vi "ZMC Open Eth.vi"(8 "error in (no error)":errorcluster caption="错误输入（无错误）", 10 "phandle":u32, 11 "ipaddr":string) -> (0 "error out":errorcluster caption="错误输出", 1 "function return":i32, 2 "phandle out":u32, 3 "ipaddr out":string)   [LabVIEW 2019, in "zauxdll.lvlib"]
doc: "int32 __stdcall ZMC_OpenEth(char *ipaddr, ZMC_HANDLE * phandle);"
uses:
  zauxdll.lvlib
  zmotion.dll
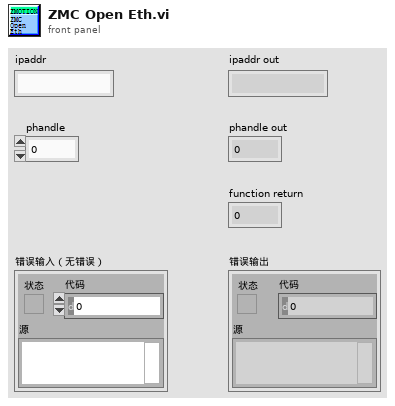
[diagram p1: front panel]
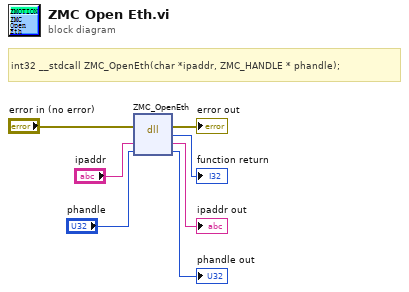
[diagram p0: block diagram]
diagram:
  # "int32 __stdcall ZMC_OpenEth(char *ipaddr, ZMC_HANDLE * phandle);"
  n1 = dll-call lib="C:/Users/VIC/Desktop/Standar Program/System/LLB/zmotion/zaux/zmotion.dll" fn="ZMC_OpenEth"(error in="error in (no error)", "ipaddr"="ipaddr", "phandle"="phandle") -> (error out=→"error out":errorcluster, "return type"=→"function return":i32, "ipaddr"=→"ipaddr out":string, "phandle"=→"phandle out":u32)  [unwired: 2 in, 1 out]
